vi "After Launch Init Core.vi"(8 "error in (no error)":errorcluster, 11 "CS++PPG in":refnum<class "CS++PPG.lvclass">) -> (0 "error out":errorcluster, 3 "CS++PPG out":refnum<class "CS++PPG.lvclass">)   [LabVIEW 2015, in "CS++PPG.lvlib" / "CS++PPG.lvclass"]
doc: "Use <b>Pre Launch init.vi</b> method for sanity checks that are supposed to prevent the actor from launching if they fail. Use <B>this</B> method instead to initialize this actor when it has been activated. A corresponding high priority message will become dispatched before the <B>Actor Core.vi</b> is called.\n\n<b>Derived classed should call the parent methode first</b> and their own initialization code after.\n\nRefer also to the ongoing discussion at https://decibel.ni.com/content/message/57394#57394."
uses:
  CS++PPG.lvclass
  CS++PPG.lvclass/CS++PPG.ctl
  CSPP_Core/Actors/CS++DeviceActor/CS++DeviceActor.lvclass
  CSPP_Core/Classes/CS++ProcessVariables/PVConnection/PVConnection.lvclass
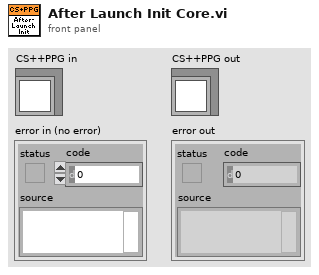
[diagram p1: front panel]
types:
  T1 = cluster{"Read Access":enum8{"Allowed", "Required", "None"}, "Write Access":enum8{"Allowed", "Required", "None"}}
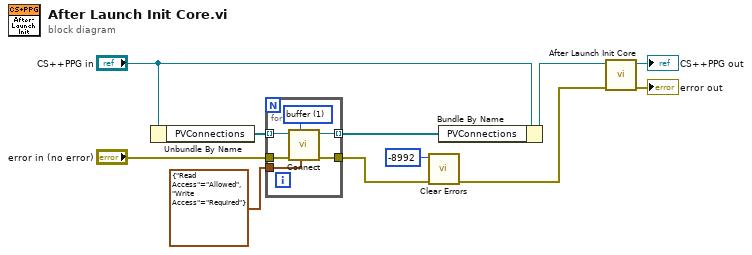
[diagram p0: block diagram]
diagram:
  n1 = Unbundle By Name("CS++PPG in") -> ("PVConnections"=w6:refnum<class "PVConnection.lvclass">[])
  n2 = for {
    tunnel: w6 -> [w17] mode=indexing
    tunnel: [w16] -> w5 mode=indexing
    tunnel: T1 {"Read Access"=enum."Allowed", "Write Access"=enum."Required"} ("Access (R/W allowed)") -> [w15]
    tunnel: [w14] -> w4
    tunnel: "error in (no error)" -> [w12]
    w13 = u16 1 items=["commit", "buffer"] ("Mode (commit)")
    n3 = call "Connect.vi"("Access (R/W allowed)"=w15, "Mode (buffer)"=w13, "Error In"=w12, "PVConnection in"=w17) -> ("Error Out"=w14:errorcluster, "PVConnection out"=w16:refnum<class "PVConnection.lvclass">)  [unwired: 6 in]
  }
  n4 = call <vilib>:"Clear Errors.vi"("error in (no error)"=w4, "specific error code to clear (0: all)"=-8992) -> ("error out"=w2:errorcluster)  [unwired: 4 in, 1 out]
  n5 = Bundle By Name(cluster="CS++PPG in", "PVConnections"=w5) -> (w8:refnum<class "CS++PPG.lvclass">)
  n6 = call-parent "After Launch Init Core.vi"("error in (no error)"=w2, "CS++DeviceActor in"=w8) -> ("error out"=→"error out":errorcluster, "CS++DeviceActor out"=→"CS++PPG out":refnum<class "CS++PPG.lvclass">)  [unwired: 8 in]
